vi "Disabled - Choose Alliance (SubVI).vi"(11 "Change Color":bool) -> (3 "Alliance Color":string)   [LabVIEW 2020]
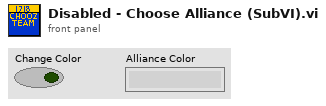
[diagram p1: front panel]
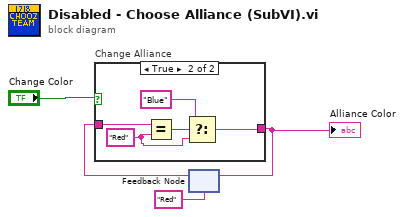
[diagram p0: block diagram]
diagram:
  n1 = feedback #1("Red") -> (w2:string)
  n2 = case "Change Alliance" shown="True" "Change Color" {
    tunnel: w2 -> [w5 w9]
    tunnel: [w5 w6] -> w4
    frame False {
    }
    frame True {
      w8 = "Red" ("x")
      n3 = Equal?(x=w9, y=w8) -> (x = y?=w10:bool)
      n4 = Select(t="Blue", s=w10, f=w8) -> (s? t:f=w6:string)
    }
  }
  "Alliance Color" <- w4
  n5 = feedback-in #1(w4) -> ()
